vi "Destructor.vi"(8 "error in (no error)":errorcluster, 11 "Mouse in":refnum<class "Joystick.lvclass">) -> (0 "error out":errorcluster)   [LabVIEW 2021, in "InputDevice.lvlib" / "Joystick.lvclass"]
uses:
  Joystick.lvclass
  <vilib>/Utility/inputDevices.llb/closeJoystick.vi
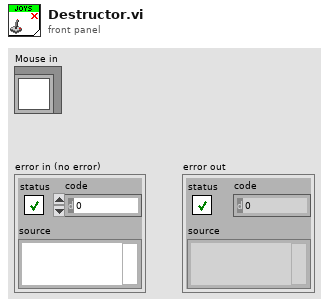
[diagram p1: front panel]
types:
  T1 = typedef "Joystick.lvclass/data.ctl" = cluster{"DeviceID":refnum<k1>, "JoyButtonInfo":refnum<user-event>, "JoyAxisInfo":refnum<user-event>, "JoyDirectionInfo":refnum<user-event>, "Joystick":refnum<event-registration>, "StopNotifier":refnum<notifier>}
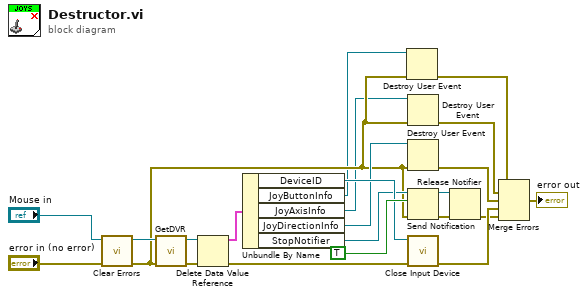
[diagram p0: block diagram]
diagram:
  n1 = call <vilib>:"Clear Errors.vi"("error in (no error)"="error in (no error)") -> ("error out"=w4:errorcluster)  [unwired: 5 in, 1 out]
  n2 = call "GetDVR.vi"("error in (no error)"=w4, "Mouse"="Mouse in") -> ("error out"=w13:errorcluster, "DVR"=w19:refnum<data-value>)  [unwired: 8 in]
  n3 = Delete Data Value Reference(data value reference=w19, error in=w13) -> (data value=w18:T1, error out=w12:errorcluster)
  n4 = Unbundle By Name(w18) -> ("DeviceID"=w17:refnum<k1>, "JoyButtonInfo"=w1:refnum<user-event>, "JoyAxisInfo"=w2:refnum<user-event>, "JoyDirectionInfo"=w11:refnum<user-event>, "StopNotifier"=w10:refnum<notifier>)
  n5 = Destroy User Event(user event=w1, error in=w4) -> (error out=w3:errorcluster)
  n6 = Destroy User Event(user event=w2, error in=w4) -> (error out=w9:errorcluster)
  n7 = Destroy User Event(user event=w11, error in=w4) -> (error out=w8:errorcluster)
  n8 = Send Notification(notification=TRUE, notifier=w10, error in (no error)=w4) -> (notifier out=w14:refnum<notifier>, error out=w15:errorcluster)
  n9 = call-poly <vilib>:"Close Input Device.vi"("error in (no error)"=w12, "device ID"=w17) -> ("error out"=w7:errorcluster)  [unwired: 8 in]
  n10 = Release Notifier(notifier=w14, error in (no error)=w15) -> (error out=w6:errorcluster)  [unwired: 1 in, 2 out]
  n11 = Merge Errors(w3, w9, w8, w7, w6) -> (→"error out":errorcluster)
